vi "Set Buffer Size.vi"(8 "error in (no error)":errorcluster, 10 "Buffer Size (#timestamps)":i32, 11 "Ring buffer DVR in":refnum<data-value>) -> (0 "error out":errorcluster, 3 "Ring buffer DVR out":refnum<data-value>)   [LabVIEW 2021, in "Ring Buffer Time Series Data.lvlib"]
uses:
  Ring Buffer Time Series Data.lvlib
  SubVIs/DVR data.ctl
  SubVIs/Split Values Array.vi
  SubVIs/Enforce array size multiple timestamps.vi
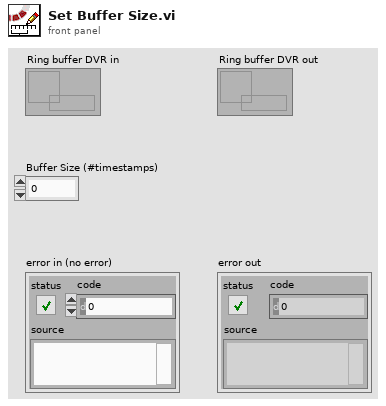
[diagram p1: front panel]
types:
  T1 = typedef "Ring Buffer Time Series Data.lvlib/DVR data.ctl" = cluster{"Timestamps":u64[], "Values":u8[], "#bytes per timestamp":i32, "Index":i32, "Size (#timestamps)":i32, "Full?":bool}
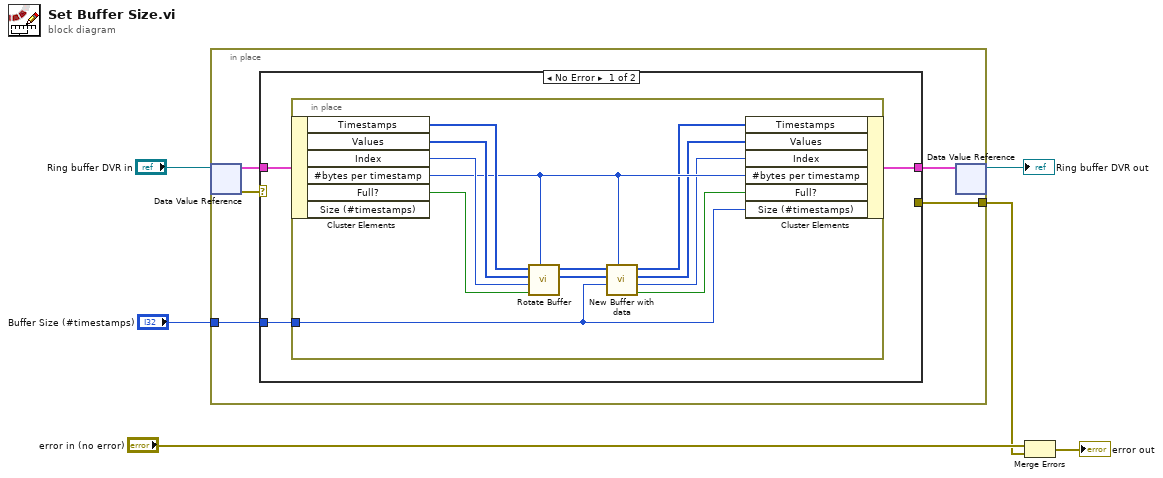
[diagram p0: block diagram]
diagram:
  n1 = in-place {
    in-place-border: [w8] -> w3
    in-place-border: "Buffer Size (#timestamps)" -> [w7]
    n2 = in-place-dvr #1("Ring buffer DVR in") -> (w10:T1, w11:errorcluster)
    n3 = case shown="No Error" w11 {
      selector: w11 -> [_ w27]
      tunnel: w10 -> [w14 _]
      tunnel: [w13 _] -> w9
      tunnel: [_ w27] -> w8
      tunnel: w7 -> [w12 _]
      frame No Error {
        n4 = in-place {
          in-place-border: w12 -> [w15]
          n5 = in-place-cluster #2(w14) -> ("Timestamps"=w26:u64[], "Values"=w25:u8[], "Index"=w24:i32, "#bytes per timestamp"=w20:i32, "Full?"=w23:bool)  [unwired: 1 out]
          n6 = call "Rotate Buffer.vi"("#bytes per value"=w20, "Full?"=w23, "Index"=w24, "Values"=w25, "Timestamps"=w26) -> ("Values"=w21:u8[], "Timestamps"=w22:u64[])  [unwired: 4 in, 1 out]
          n7 = call "New Buffer with data.vi"("#bytes per timestamp"=w20, "New Buffer Size (#timestamps)"=w15, "Values (buffered, rotated)"=w21, "Timestamps (buffered, rotated)"=w22) -> ("Full?"=w16:bool, "index"=w17:i32, "Values (new buffer)"=w18:u8[], "Timestamps (new buffer)"=w19:u64[])  [unwired: 4 in]
          n8 = in-place-cluster #2("Timestamps"=w19, "Values"=w18, "Index"=w17, "#bytes per timestamp"=w20, "Full?"=w16, "Size (#timestamps)"=w15) -> (w13:T1)
        }
      }
      frame Error {
      }
    }
    n9 = in-place-dvr #1(w9) -> (→"Ring buffer DVR out":refnum<data-value>)  [unwired: 1 out]
  }
  n10 = Merge Errors("error in (no error)", w3) -> (→"error out":errorcluster)
